vi "Actuate Digital Line.vi"(6 "Simulate":bool, 8 "error in":errorcluster, 9 "timeout":dbl=10.0 format="%0.2f", 10 "state":bool, 11 "DO-Line Ref":refnum<k21>) -> (0 "error out":errorcluster, 3 "DO-Line Ref out":refnum<k21>)   [LabVIEW 2017, in "DAQ.lvclass"]
doc: "Developed by Kevin Thompson\nThompson Engineering, LLC\nkevin@thompsonengineering.net"
uses:
  DAQ.lvclass
  <vilib>/DAQmx/write.llb/DAQmx Write (Digital Bool 1Line 1Point).vi
  <vilib>/DAQmx/miscellaneous.llb/DAQmx Fill In Error Info.vi
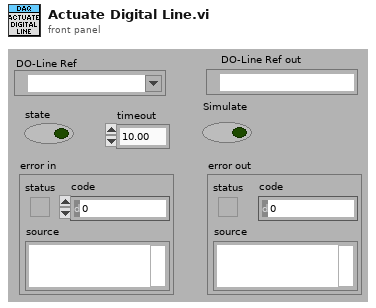
[diagram p1: front panel]
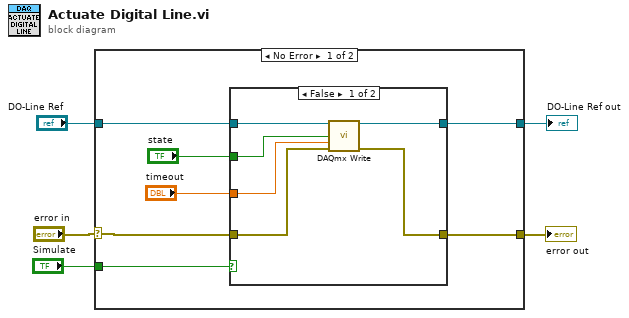
[diagram p0: block diagram]
diagram:
  n1 = case shown="No Error" "error in" {
    selector: "error in" -> [w7 w21]
    tunnel: "DO-Line Ref" -> [w12 w22]
    tunnel: [w11 w22] -> w4
    tunnel: [w10 w21] -> w3
    tunnel: "Simulate" -> [w6 _]
    frame No Error {
      n2 = case shown="False" w6 {
        tunnel: w12 -> [w18 w20]
        tunnel: [w17 w20] -> w11
        tunnel: [w16 w19] -> w10
        tunnel: "state" -> [w15 _]
        tunnel: "timeout" -> [w14 _]
        tunnel: w7 -> [w13 w19]
        frame False {
          n3 = call-poly <vilib>:"DAQmx Write.vi"("task/channels in"=w18, "data"=w15, "timeout"=w14, "error in"=w13) -> ("task out"=w17:refnum<k21>, "error out"=w16:errorcluster)  [unwired: 9 in, 1 out]
        }
        frame True {
        }
      }
    }
    frame Error {
    }
  }
  "error out" <- w3
  "DO-Line Ref out" <- w4
